vi "project3drafting.vi"() -> ()   [LabVIEW 2022 SP3]
uses:
  <vilib>/MakerHub/LINX/Public/Peripherals/Digital/Digital Write 1 Chan.vi
  <vilib>/Analysis/baseanly.llb/Mean (DBL).vi
  <vilib>/Analysis/2dsp.llb/1D Auto Correlation (DBL).vi
  <vilib>/MakerHub/LINX/Public/Peripherals/Digital/Digital Write N Chans.vi
  <vilib>/MakerHub/LINX/Private/Local IO/LinxDigitalWrite.vi
  <vilib>/MakerHub/LINX/Public/Utilities/Check Channel.vi
  <vilib>/MakerHub/LINX/Public/Utilities/Open Serial.vi
  <vilib>/MakerHub/LINX/Private/Utilties/Generate Error.vi
  <vilib>/Analysis/NI_AALBase.lvlib
  <vilib>/MakerHub/LINX/LMH-LINX.lvlib
  <vilib>/Analysis/NI_AALPro.lvlib
  <vilib>/Analysis/NI_AAL_SigProc.lvlib
panel:
  in  "led output pin":u16
  in  "Serial Port":refnum<visa-resource-name>="N/A"
  out "BPM":dbl
  out "Peaks found":i32
  in  "Peaks width":i32=3 min=3
  in  "Peaks threshold":dbl format="%0.2f"
  out "Right Side Autocorrelation":dbl[](graph)
  out "Filtered and Normalized Waveform":waveform(dbl)(graph)
  out "Raw Waveform":waveform(dbl)(graph)
  in  "waiting seconds for saving":i32
  out "Loop Rate (Hz)":u32
  in  "stop":bool
  in  "Sampling duration (s)":dbl
  in  "Sampling freq (Hz)":dbl
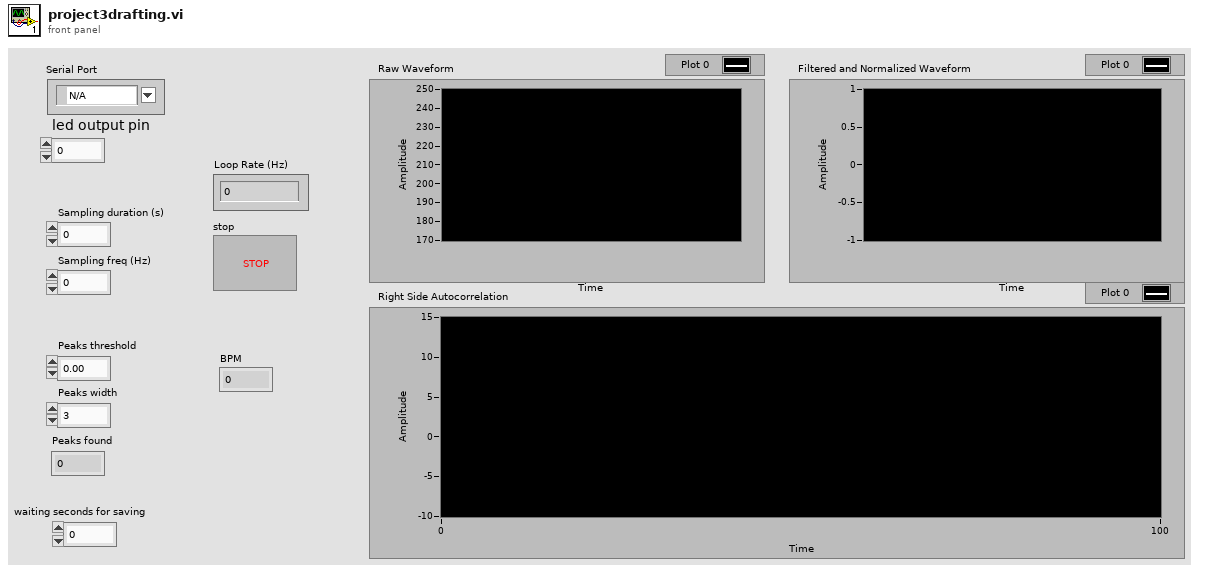
[diagram p1: front panel]
types:
  T1 = typedef "LMH-LINX.lvlib/LINX Ref.ctl" = cluster{"IO":T2, "Interface":T3, "LINX Device Config":T4}
  T2 = typedef "LMH-LINX.lvlib/Platform.ctl" = enum16{"Remote", "Local"}
  T3 = typedef "LMH-LINX.lvlib/Interface.ctl" = enum16{"Serial", "TCP"}
  T4 = typedef "LMH-LINX.lvlib/Device.lvlib/LINX Device Config.ctl" = cluster{"Interface":T3, "COM Port":refnum<visa-resource-name>, "TCP Configuration":T5, "Device Family":u8, "Device ID":u8, "Device Name":string, "TCP Ref":refnum<k5>, "Channels":T6}
  T5 = typedef "LMH-LINX.lvlib/Device.lvlib/TCP Config.ctl" = cluster{"IP Address":string, "Port":u16}
  T6 = typedef "LMH-LINX.lvlib/Channels.ctl" = cluster{"DI":u8[], "DO":u8[], "AI":u8[], "AO":u8[], "PWM":u8[], "QE":u8[], "UART":u8[], "I2C 2":u8[], "SPI":u8[], "CAN":u8[], "Servo":u8[], "AI Ref (V)":dbl, "AI Resolution (Bits)":u8, "AO Ref (V)":dbl, "AO Resolution (Bits)":u8}
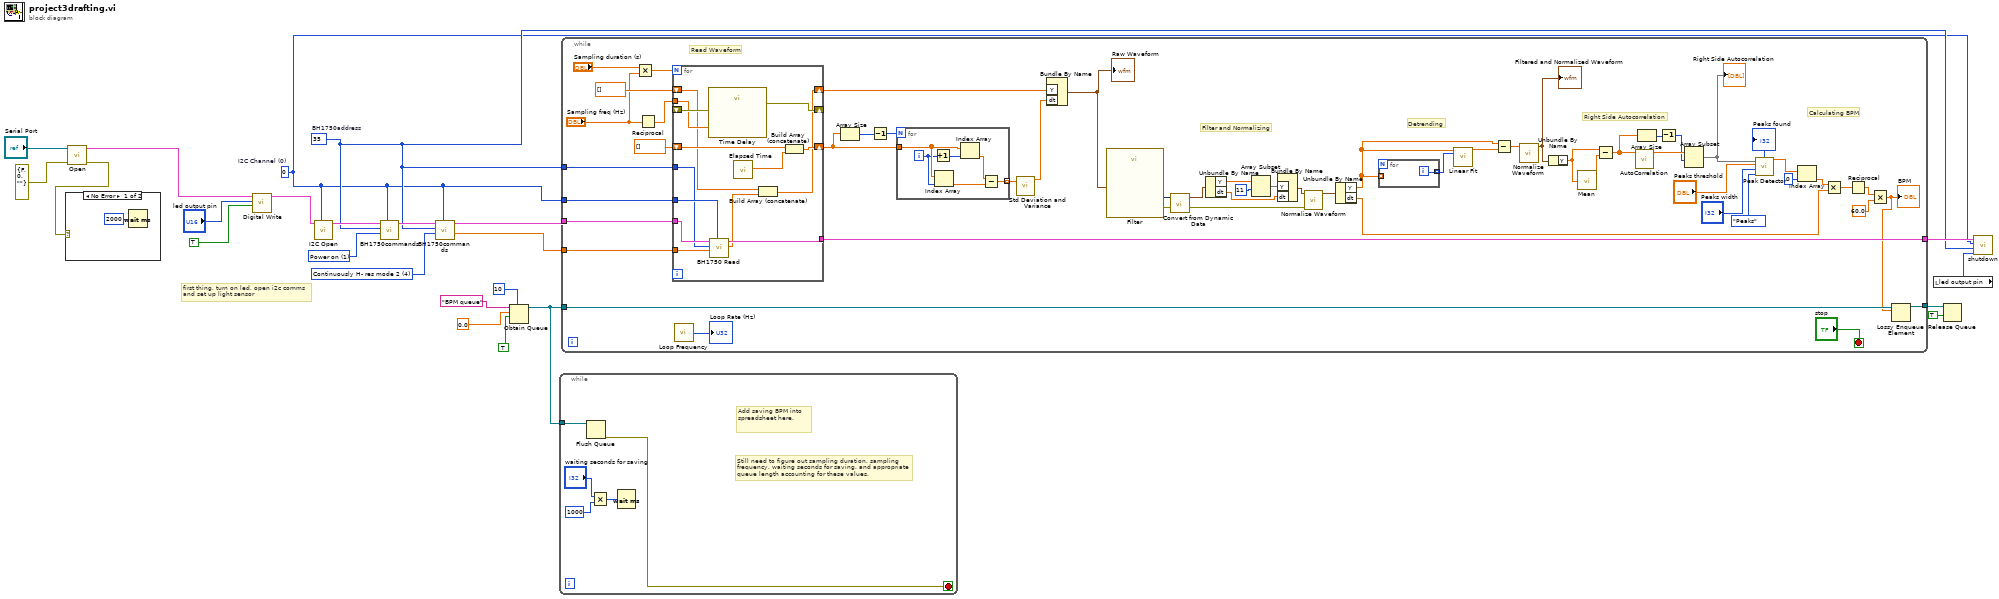
[diagram p0: block diagram]
diagram:
  w7 = u16 4 items=["power down", "Power on", "Reset", "Continuously H- res", "Continuously H- res mode 2", "Continuously L- res", "One time H- res ", "One time H- res mode 2", "One time L res ", "Change Measurement time High bit", "Change Measurement time  Low Bit"] ("Command")
  w9 = u16 1 items=["power down", "Power on", "Reset", "Continuously H- res", "Continuously H- res mode 2", "Continuously L- res", "One time H- res ", "One time H- res mode 2", "One time L res ", "Change Measurement time High bit", "Change Measurement time  Low Bit"] ("Command")
  w3 = u8 35  # BH1750address
  w2 = u8 0  # I2C Channel (0)
  # "first thing, turn on led, open i2c comms\nand set up light sensor"
  n1 = call-poly <vilib>:"Open.vi"("Error In"=errorcluster {"status"=FALSE, "code"=0, "source"=""}, "Serial Port"="Serial Port") -> ("Error Out"=w12:errorcluster, "LINX Resource"=w15:T1)  [unwired: 7 in, 1 out]
  n2 = case shown="No Error" w12 {
    frame No Error {
      n3 = Wait (ms)(milliseconds to wait=u32 2000) -> ()  [unwired: 1 out]
    }
    frame Error {
    }
  }
  n4 = call-poly <vilib>:"Digital Write.vi"("Output Value"=TRUE, "DO Channel"="led output pin", "LINX Resource"=w15) -> ("LINX Resource"=w11:T1)  [unwired: 7 in, 1 out]
  n5 = call <vilib>:"I2C Open.vi"("I2C Channel (0)"=w2, "LINX Resource"=w11) -> ("LINX Resource"=w10:T1)  [unwired: 8 in, 1 out]
  n6 = call "BH1750commands.vi"("I2C Channel"=w2, "Command"=w9, "I2C Slave Address (0)"=w3, "LINX Resource"=w10) -> ("LINX Resource out"=w8:T1)  [unwired: 5 in, 2 out]
  n7 = call "BH1750commands.vi"("I2C Channel"=w2, "Command"=w7, "I2C Slave Address (0)"=w3, "LINX Resource"=w8) -> ("Resoultion (lux)"=w5:dbl, "LINX Resource out"=w6:T1)  [unwired: 5 in, 1 out]
  n8 = Obtain Queue(max queue size (-1, unlimited)=10, name (unnamed)="BPM queue", element data type=0.0, create if not found? (T)=TRUE) -> (queue out=w19:refnum<queue>)  [unwired: 1 in, 2 out]
  n9 = while {
    tunnel: w19 -> [w27]
    stop <- w26 stop-if-true
    # "Still need to figure out sampling duration, sampling \nfrequency, waiting seconds for saving, and appropriate \nqueue length accounting for these values."
    # "Add saving BPM into spreadsheet here."
    n10 = Flush Queue(queue=w27) -> (error out=w26:errorcluster)  [unwired: 1 in, 2 out]
    n11 = Multiply(x="waiting seconds for saving", y=1000) -> (x*y=w30:i32)
    n12 = Wait (ms)(milliseconds to wait=w30) -> ()  [unwired: 1 out]
  }
  n13 = while {
    tunnel: w6 -> [w73]
    tunnel: [w72] -> w4
    tunnel: w19 -> [w70]
    tunnel: [w69] -> w21
    tunnel: w2 -> [w33]
    tunnel: w5 -> [w32]
    tunnel: w3 -> [w31]
    stop <- "stop" stop-if-true
    # "Calculating BPM"
    # "Right Side Autocorrelation"
    # "Detrending"
    # "Filter and Normalizing"
    # "Read Waveform"
    n14 = Multiply(x="Sampling duration (s)", y="Sampling freq (Hz)") -> (x*y=w78:dbl)
    n15 = Reciprocal(x="Sampling freq (Hz)") -> (1/x=w74:dbl)
    n16 = for {
      N: w78 -> [_]
      tunnel: w73 -> [w99]
      shift-right: [w106] -> _
      shift-left: _ -> [w107]
      tunnel: w74 -> [w105]
      shift-right: [w102] -> w79
      shift-left: dbl[] [] -> [w103]
      tunnel: [w95] -> w72
      shift-right: [w101] -> w84
      shift-left: dbl[] [] -> [w100]
      tunnel: w33 -> [w98]
      tunnel: w32 -> [w97]
      tunnel: w31 -> [w96]
      n17 = call "Time Delay"("error in (no error)"=w107, "Delay Time (s)"=w105) -> ("error out"=w106:errorcluster)  [unwired: 9 in]
      n18 = call "BH1750 Read.vi"("I2C Channel (0)"=w98, "Resoultion (lux)"=w97, "BH1750address"=w96, "LINX Resource in"=w99) -> ("Lux value"=w94:dbl, "LINX Resource"=w95:T1)  [unwired: 4 in, 2 out]
      n19 = call "Elapsed Time"() -> ("Elapsed Time (s)"=w104:dbl)  [unwired: 12 in, 7 out]
      n20 = Build Array (concatenate)(w100, w94) -> (w101:dbl[])
      n21 = Build Array (concatenate)(w103, w104) -> (w102:dbl[])
    }
    n22 = call <vilib>:"Loop Frequency.vi"() -> ("Loop Rate (Hz)"=→"Loop Rate (Hz)":u32)
    n23 = Array Size(array=w79) -> (size(s)=w80:i32)
    n24 = Decrement(x=w80) -> (x-1=w81:i32)
    n25 = for {
      N: w81 -> [_]
      tunnel: w79 -> [w93]
      tunnel: [w88] -> w82 mode=indexing
      i -> [w91]
      n26 = Increment(x=w91) -> (x+1=w92:i32)
      n27 = Index Array(array=w93, index=w91) -> (element=w89:dbl)
      n28 = Index Array(array=w93, index=w92) -> (element=w90:dbl)
      n29 = Subtract(x=w90, y=w89) -> (x-y=w88:dbl)
    }
    n30 = call <vilib>:"Std Deviation and Variance.vi"("X"=w82) -> ("mean"=w85:dbl)  [unwired: 1 in, 2 out]
    n31 = Bundle By Name("Y"=w84, "dt"=w85) -> (w67:waveform(dbl))  [unwired: 1 in]
    "Raw Waveform" <- w67
    n32 = call "Filter"("Signal"=w67) -> ("error out"=w49:errorcluster, "Filtered Signal"=w61:dynamicdata)  [unwired: 9 in]
    n33 = call "Convert from Dynamic Data"("Dynamic Data Type"=w61) -> ("Waveform"=w66:waveform(dbl))  [unwired: 3 in]
    n34 = Unbundle By Name(w66) -> ("Y"=w65:dbl[], "dt"=w62:dbl)
    n35 = Array Subset(array=w65, index=11) -> (w63:dbl[])  [unwired: 1 in]
    n36 = Bundle By Name("Y"=w63, "dt"=w62) -> (w47:waveform(dbl))  [unwired: 1 in]
    n37 = call <vilib>:"Normalize Waveform.vi"("error in (no error)"=w49, "waveform in"=w47) -> ("normalized waveform"=w48:waveform(dbl))  [unwired: 6 in, 3 out]
    n38 = Unbundle By Name(w48) -> ("Y"=w59:dbl[], "dt"=w38:dbl)
    n39 = for {
      tunnel: [w87] -> w60 mode=indexing
      tunnel: [w86] -> _ mode=indexing
      tunnel: w59 -> [w86] mode=indexing
      i -> [w87]
    }
    n40 = call <vilib>:"Linear Fit.vi"("Y"=w59, "X"=w60) -> ("Best Linear Fit"=w58:dbl[])  [unwired: 9 in, 4 out]
    n41 = Subtract(x=w59, y=w58) -> (x-y=w57:dbl[])
    n42 = call <vilib>:"Normalize Waveform.vi"("waveform in"=w57) -> ("normalized waveform"=w56:waveform(dbl))  [unwired: 7 in, 3 out]
    "Filtered and Normalized Waveform" <- w56
    n43 = Unbundle By Name(w56) -> ("Y"=w54:dbl[])
    n44 = call-poly <vilib>:"Mean.vi"("X"=w54) -> ("mean"=w55:dbl)  [unwired: 1 out]
    n45 = Subtract(x=w54, y=w55) -> (x-y=w53:dbl[])
    n46 = call-poly <vilib>:"AutoCorrelation.vi"("X"=w53) -> ("Rxx"=w51:dbl[])  [unwired: 9 in, 1 out]
    n47 = Array Size(array=w53) -> (size(s)=w52:i32)
    n48 = Decrement(x=w52) -> (x-1=w50:i32)
    n49 = Array Subset(array=w51, index=w50) -> (w46:dbl[])  [unwired: 1 in]
    "Right Side Autocorrelation" <- w46
    n50 = call <vilib>:"Peak Detector.vi"("peaks/valleys"=enum32{"Peaks", "Valleys"}."Peaks", "width"="Peaks width", "threshold"="Peaks threshold", "X"=w46) -> ("Locations"=w41:dbl[], "# found"=→"Peaks found":i32)  [unwired: 3 in, 3 out]
    n51 = Index Array(array=w41, index=0) -> (element=w39:dbl)
    n52 = Multiply(x=w39, y=w38) -> (x*y=w37:dbl)
    n53 = Reciprocal(x=w37) -> (1/x=w36:dbl)
    n54 = Multiply(x=w36, y=60.0) -> (x*y=w34:dbl)
    "BPM" <- w34
    n55 = Lossy Enqueue Element(queue=w70, element=w34) -> (queue out=w69:refnum<queue>)  [unwired: 1 in, 3 out]
  }
  n56 = local read "led output pin"() -> (w1:u16)
  n57 = Release Queue(queue=w21, force destroy? (F)=TRUE) -> ()  [unwired: 1 in, 3 out]
  n58 = call "shutdown.vi"("LINX Resource"=w4, "I2C channel wire"=w2, "BH1750 address wire"=w3, "led output pin"=w1) -> ()  [unwired: 7 in]
